vi "SetParam.vi"(8 "error in (no error)":errorcluster caption="entrée d'erreur (pas d'erreur)", 10 "Nystroem":T1={"kernel"="rbf", "gamma"="None", "coef0"="None", "degree"="None", "kernel_params"="None", "n_components"=100, "random_state"=-1} {"random_state" min=-1}, 11 "Nystroem.lvclass":refnum<class "Nystroem.lvclass">) -> (0 "error in (no error)":errorcluster caption="entrée d'erreur (pas d'erreur)", 3 "Nystroem.lvclass":refnum<class "Nystroem.lvclass">)   [LabVIEW 2020, in "Nystroem.lvclass"]
doc: "Set Parameters"
uses:
  Nystroem.lvclass
  Nystroem.lvclass/Nystroem.ctl
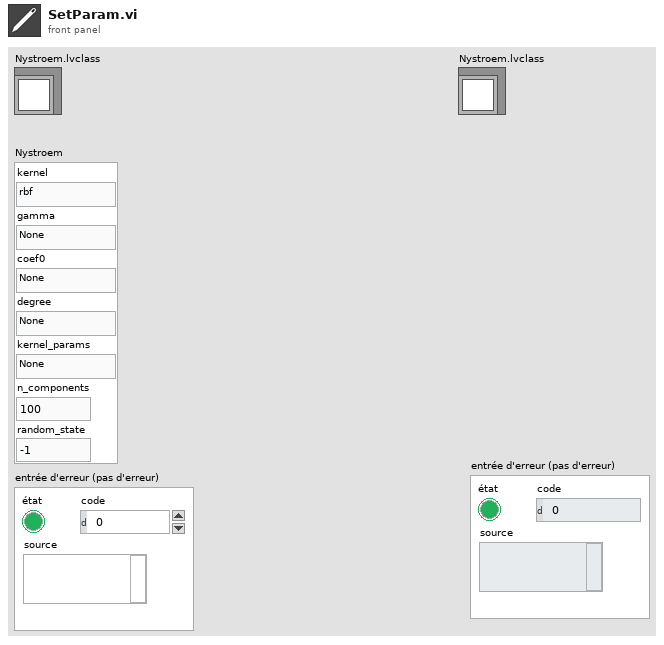
[diagram p1: front panel]
types:
  T1 = cluster{"kernel":string, "gamma":string, "coef0":string, "degree":string, "kernel_params":string, "n_components":i32, "random_state":i32}
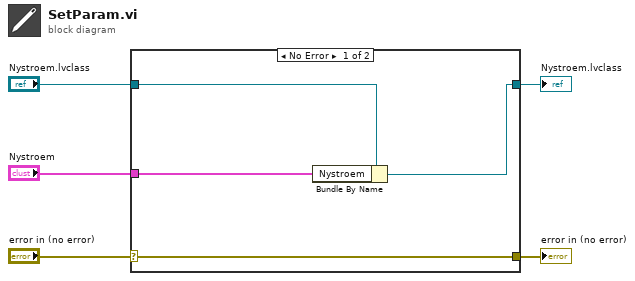
[diagram p0: block diagram]
diagram:
  n1 = case shown="No Error" "error in (no error)" {
    selector: "error in (no error)" -> [w9 w10]
    tunnel: [w9 w10] -> w4
    tunnel: [w7 w11] -> w2
    tunnel: "Nystroem.lvclass" -> [w8 w11]
    tunnel: "Nystroem" -> [w6 _]
    frame No Error {
      n2 = Bundle By Name(cluster=w8, "Nystroem"=w6) -> (w7:refnum<class "Nystroem.lvclass">)
    }
    frame Error {
    }
  }
  "error in (no error)" <- w4
  "Nystroem.lvclass" <- w2
